vi "subvi_dc_motor_pwm.vi"(10 "Duty Cycle (%)":sgl, 11 "Frequency (Hz)":sgl) -> (2 "Wait time":sgl, 3 "Cycle time":sgl)   [LabVIEW 2019]
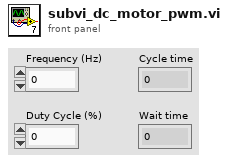
[diagram p1: front panel]
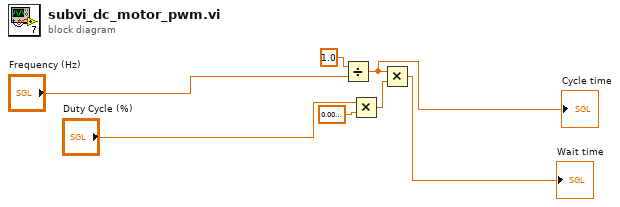
[diagram p0: block diagram]
diagram:
  n1 = Divide(x=sgl 1.0 ("Frequency (Hz)) 2"), y="Frequency (Hz)") -> (x/y=w7:sgl)
  "Cycle time" <- w7
  n2 = Multiply(x="Duty Cycle (%)", y=sgl 0.01) -> (x*y=w4:sgl)
  n3 = Multiply(x=w7, y=w4) -> (x*y=→"Wait time":sgl)
